vi "Obtain Queue.vi"(8 "error in (no error)":errorcluster, 9 "Region":T1, 10 "Name":string, 11 "AWS Credentials":T2) -> (0 "error out":errorcluster, 3 "SQS":refnum<class "Queue.lvclass">)   [LabVIEW 2015, in "NI_AWS_SQS.lvlib" / "Queue.lvclass"]
doc: "Returns an existing queue. This action provides a simple way to retrieve the Amazon SQS queue."
uses:
  Queue.lvclass
  Core/HTTP Request/AWS Credentials.ctl
  Core/HTTP Request/Region.ctl
  Queue.lvclass/Queue.ctl
  Read Name.vi
  Core/HTTP Request/HTTP Request.lvclass
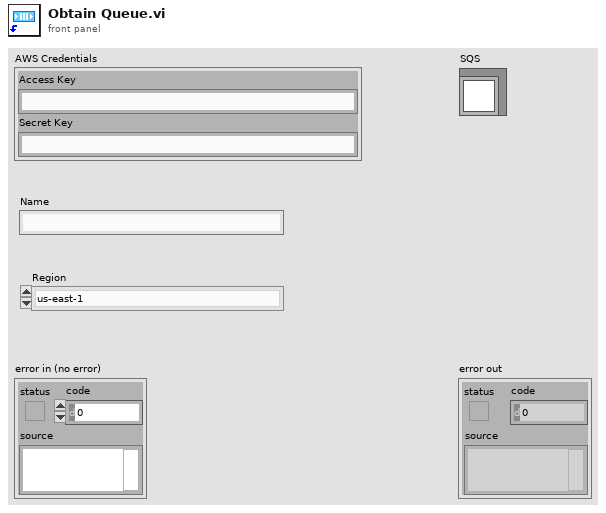
[diagram p1: front panel]
types:
  T1 = typedef "NI_AWS_Core.lvlib/HTTP Request.lvclass/Region.ctl" = enum16{"us-east-1", "us-east-2", "us-west-1", "us-west-2", "ap-northeast-1", "ap-northeast-2", "ap-southeast-1", "ap-southeast-2", "ca-central-1", "eu-central-1", "eu-west-1", "eu-west-2", "sa-east-1"}
  T2 = typedef "NI_AWS_Core.lvlib/HTTP Request.lvclass/AWS Credentials.ctl" = cluster{"Access Key":string, "Secret Key":string}
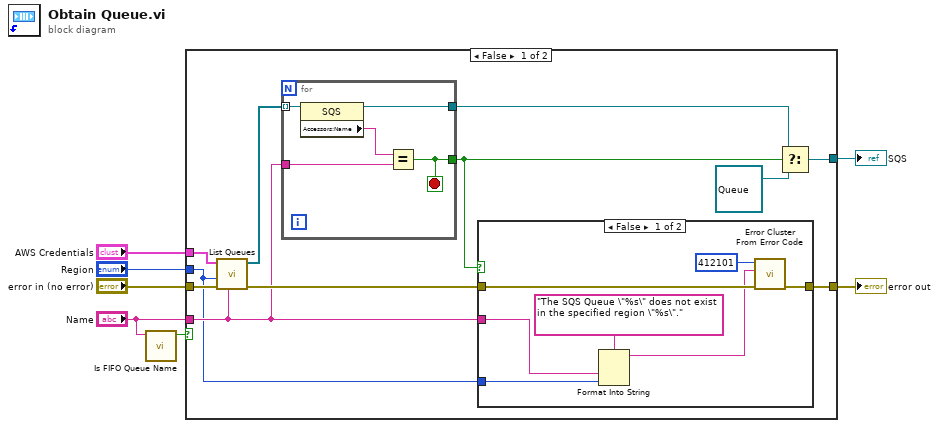
[diagram p0: block diagram]
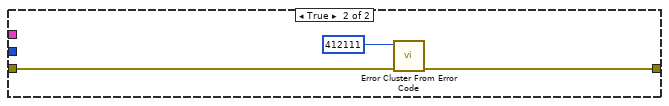
[diagram p3: hidden frame]
diagram:
  n1 = call "Is FIFO Queue Name.vi"("Name"="Name") -> ("FIFO Queue"=w1:bool)  [unwired: 10 in]
  n2 = case shown="False" w1 {
    tunnel: "error in (no error)" -> [w18 w33]
    tunnel: "AWS Credentials" -> [w17 _]
    tunnel: "Region" -> [w8 _]
    tunnel: [w13 _] -> w4
    tunnel: [w10 w32] -> w3
    tunnel: "Name" -> [w9 _]
    frame False {
      n3 = call "List Queues.vi"("Name Prefix"=w9, "error in (no error)"=w18, "Region"=w8, "AWS Credentials"=w17) -> ("error out"=w11:errorcluster, "SQS Queues"=w16:refnum<class "Queue.lvclass">[])  [unwired: 6 in]
      n4 = for {
        tunnel: w16 -> [w23] mode=indexing
        tunnel: w9 -> [w21]
        tunnel: [w20] -> w12
        tunnel: [w19] -> w15
        stop <- w20 stop-if-true
        n5 = property class="SQS"(reference=w23) -> (reference out=w19:refnum<class "Queue.lvclass">, "Accessors:Name"=w22:string)  [unwired: 1 in, 1 out]
        n6 = Equal?(x=w22, y=w21) -> (x = y?=w20:bool)
      }
      n7 = case shown="False" w12 {
        tunnel: w11 -> [w30 w31]
        tunnel: [w29 w31] -> w10
        tunnel: w9 -> [w25 _]
        tunnel: w8 -> [w24 _]
        frame False {
          n8 = Format Into String(format string="The SQS Queue \"%s\" does not exist in the specified region \"%s\".", w25, w24) -> (resulting string=w26:string)  [unwired: 2 in, 1 out]
          n9 = call <vilib>:"Error Cluster From Error Code.vi"("error in (no error)"=w30, "error message (\"\")"=w26, "error code (0)"=412101) -> ("error out"=w29:errorcluster)  [unwired: 6 in]
        }
        frame True {
        }
      }
      n10 = Select(t=w15, s=w12, f=refnum<class "Queue.lvclass"> refnum ("NI_SQS.lvlib:SQS")) -> (s? t:f=w13:refnum<class "Queue.lvclass">)
    }
    frame True {
      n11 = call <vilib>:"Error Cluster From Error Code.vi"("error in (no error)"=w33, "error code (0)"=412111) -> ("error out"=w32:errorcluster)  [unwired: 7 in]
    }
  }
  "error out" <- w3
  "SQS" <- w4
